vi "Posterior_LDA_maker.vi"(2 "Target_LDA_Parameter":dbl[][](array[numeric]), 3 "Nontarget_LDA_Parameter":dbl[][](array[numeric])) -> (0 "A * B 2":T1 caption="A * B(Point)", 1 "A * B":T1 caption="A * B(Matrix)")   [LabVIEW 2013]
uses:
  <vilib>/Analysis/Matrix/Datatypes/RealMatrix.ctl
  <vilib>/Analysis/baseanly.llb/Mean (DBL).vi
  <vilib>/Analysis/baseanly.llb/Real A x B.vi
  <vilib>/Analysis/7linalg.llb/Real Transpose Matrix.vi
  <vilib>/Analysis/Matrix/Numeric/Conversions/Array To Matrix - RA2.vi
  <vilib>/Analysis/Matrix/Numeric/Multiply/Multiply - RM,R.vi
  <vilib>/Analysis/Matrix/Numeric/Add/Add - RM,RM.vi
  <vilib>/Analysis/baseanly.llb/Real Inverse Matrix.vi
  <vilib>/Analysis/Matrix/Numeric/Conversions/Array To Matrix - RA.vi
  <vilib>/Analysis/Matrix/Numeric/Subtract/Subtract - RM,RM.vi
  <vilib>/Analysis/Matrix/Numeric/Multiply/Multiply - R,RM.vi
  <vilib>/Analysis/Matrix/Numeric/Multiply/Multiply - RM,RM.vi
  <vilib>/Analysis/NI_AALBase.lvlib
  <vilib>/Analysis/Matrix/NI_Matrix.lvlib
  <vilib>/Analysis/NI_AALPro.lvlib
panel:
  out "Array":dbl[](array[numeric])
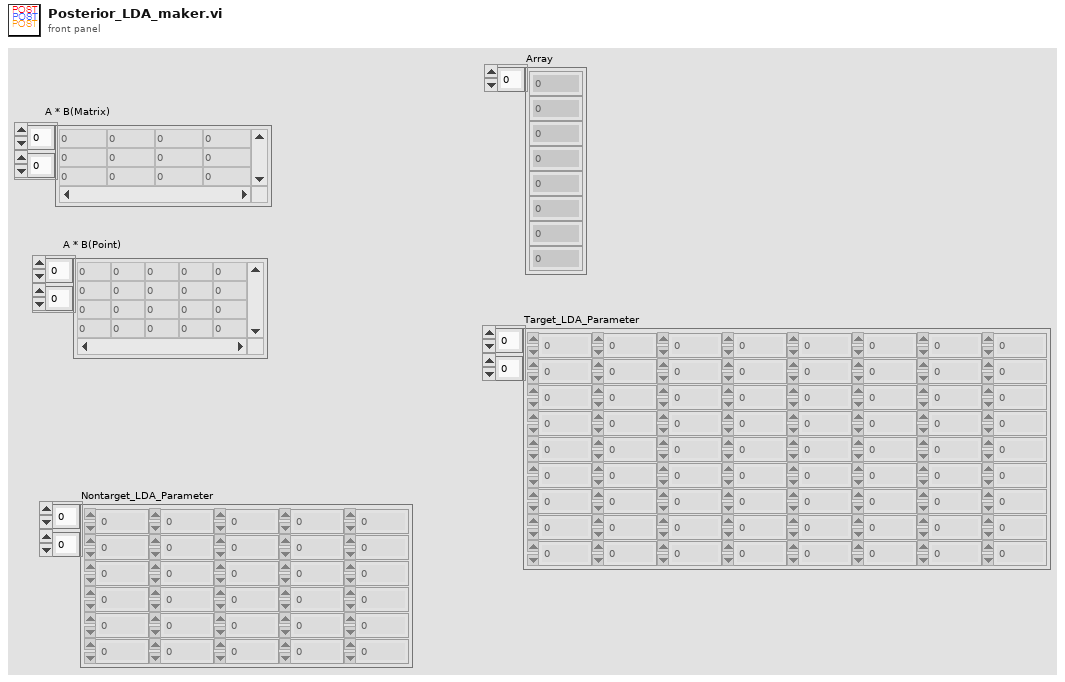
[diagram p1: front panel]
types:
  T1 = typedef "NI_Matrix.lvlib/RealMatrix.ctl" = dbl[][]
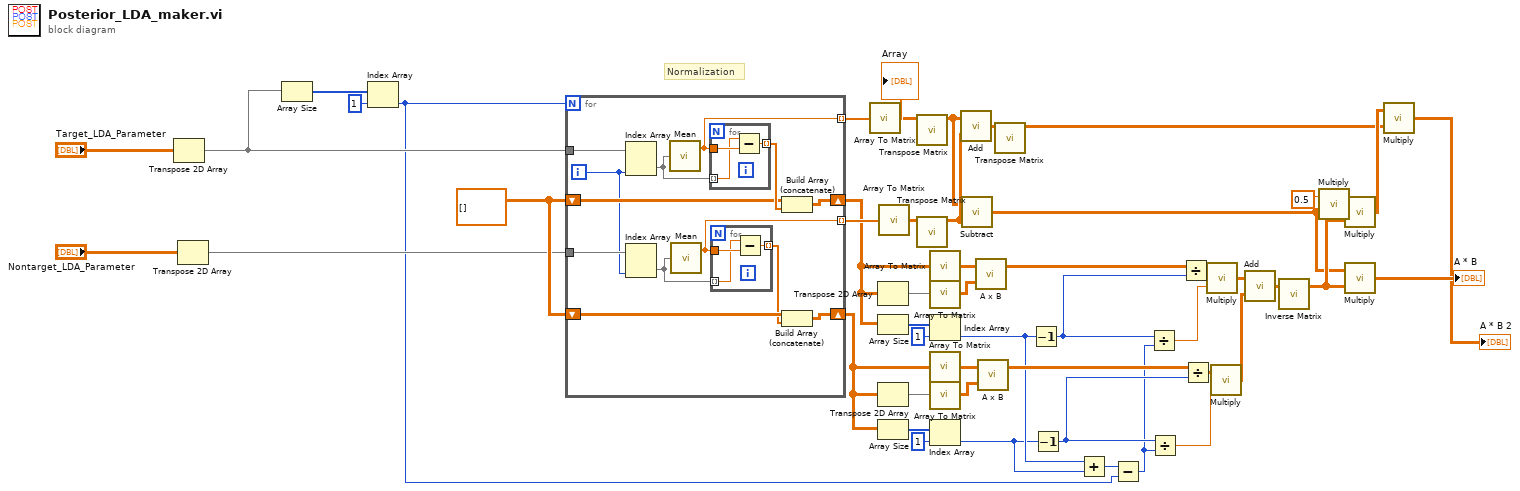
[diagram p0: block diagram]
diagram:
  w49 = dbl[][] []
  # "Normalization"
  n1 = Transpose 2D Array(2D array="Target_LDA_Parameter") -> (transposed array=w3:dbl[][])
  n2 = Transpose 2D Array(2D array="Nontarget_LDA_Parameter") -> (transposed array=w2:dbl[][])
  n3 = Array Size(array=w3) -> (size(s)=w5:i32[])
  n4 = Index Array(array=w5, index=1) -> (element=w1:i32)
  n5 = for {
    N: w1 -> [_]
    shift-right: [w62] -> w36
    shift-left: w49 -> [w61]
    shift-right: [w59] -> w34
    shift-left: w49 -> [w60]
    tunnel: [w57] -> w48 mode=indexing
    tunnel: [w56] -> w47 mode=indexing
    tunnel: w3 -> [w55]
    tunnel: w2 -> [w54]
    i -> [w51]
    n6 = Index Array(array=w55, index (col)=w51) -> (element=w53:dbl[])  [unwired: 1 in]
    n7 = Index Array(array=w54, index (col)=w51) -> (element=w52:dbl[])  [unwired: 1 in]
    n8 = call-poly <vilib>:"Mean.vi"("X"=w53) -> ("mean"=w57:dbl)  [unwired: 1 out]
    n9 = call-poly <vilib>:"Mean.vi"("X"=w52) -> ("mean"=w56:dbl)  [unwired: 1 out]
    n10 = for {
      tunnel: w57 -> [w69]
      tunnel: [w68] -> w63 mode=indexing
      tunnel: w53 -> [w67] mode=indexing
      n11 = Subtract(x=w67, y=w69) -> (x-y=w68:dbl)
    }
    n12 = for {
      tunnel: w56 -> [w66]
      tunnel: [w65] -> w58 mode=indexing
      tunnel: w52 -> [w64] mode=indexing
      n13 = Subtract(x=w64, y=w66) -> (x-y=w65:dbl)
    }
    n14 = Build Array (concatenate)(w61, w63) -> (w62:dbl[][])
    n15 = Build Array (concatenate)(w60, w58) -> (w59:dbl[][])
  }
  "Array" <- w48
  n16 = call-poly <vilib>:"Array To Matrix.vi"("Real 1D Array"=w48) -> ("Real Matrix (Column Vector)"=w46:T1)
  n17 = Transpose 2D Array(2D array=w36) -> (transposed array=w37:dbl[][])
  n18 = Array Size(array=w36) -> (size(s)=w38:i32[])
  n19 = Transpose 2D Array(2D array=w34) -> (transposed array=w35:dbl[][])
  n20 = Array Size(array=w34) -> (size(s)=w41:i32[])
  n21 = call-poly <vilib>:"Array To Matrix.vi"("Real 1D Array"=w47) -> ("Real Matrix (Column Vector)"=w45:T1)
  n22 = call-poly <vilib>:"Transpose Matrix.vi"("Input Matrix"=w46) -> ("Matrix Transpose"=w43:T1)  [unwired: 9 in, 1 out]
  n23 = call-poly <vilib>:"Transpose Matrix.vi"("Input Matrix"=w45) -> ("Matrix Transpose"=w44:T1)  [unwired: 9 in, 1 out]
  n24 = call-poly <vilib>:"Array To Matrix.vi"("Real 2D Array"=w36) -> ("Real Matrix"=w33:T1)
  n25 = call-poly <vilib>:"Array To Matrix.vi"("Real 2D Array"=w37) -> ("Real Matrix"=w32:T1)
  n26 = Index Array(array=w38, index=1) -> (element=w27:i32)
  n27 = call-poly <vilib>:"Array To Matrix.vi"("Real 2D Array"=w34) -> ("Real Matrix"=w31:T1)
  n28 = call-poly <vilib>:"Array To Matrix.vi"("Real 2D Array"=w35) -> ("Real Matrix"=w30:T1)
  n29 = Index Array(array=w41, index=1) -> (element=w26:i32)
  n30 = call-poly <vilib>:"Add.vi"("Real Matrix B"=w44, "Real Matrix A"=w43) -> ("A + B"=w42:T1)
  n31 = call-poly <vilib>:"Subtract.vi"("Real Matrix B"=w44, "Real Matrix A"=w43) -> ("A - B"=w7:T1)
  n32 = call-poly <vilib>:"A x B.vi"("B"=w32, "A"=w33) -> ("A x B"=w29:T1)  [unwired: 1 out]
  n33 = call-poly <vilib>:"A x B.vi"("B"=w30, "A"=w31) -> ("A x B"=w28:T1)  [unwired: 1 out]
  n34 = call-poly <vilib>:"Transpose Matrix.vi"("Input Matrix"=w42) -> ("Matrix Transpose"=w8:T1)  [unwired: 9 in, 1 out]
  n35 = Decrement(x=w27) -> (x-1=w24:i32)
  n36 = Decrement(x=w26) -> (x-1=w23:i32)
  n37 = Add(x=w27, y=w26) -> (x+y=w25:i32)
  n38 = Subtract(x=w25, y=w1) -> (x-y=w22:i32)
  n39 = Divide(x=w24, y=w22) -> (x/y=w20:dbl)
  n40 = Divide(x=w23, y=w22) -> (x/y=w18:dbl)
  n41 = Divide(x=w29, y=w24) -> (x/y=w21:T1)
  n42 = Divide(x=w28, y=w23) -> (x/y=w19:T1)
  n43 = call-poly <vilib>:"Multiply.vi"("Real Scalar c"=w20, "Real Matrix A"=w21) -> ("A * c"=w17:T1)
  n44 = call-poly <vilib>:"Multiply.vi"("Real Scalar c"=w18, "Real Matrix A"=w19) -> ("A * c"=w16:T1)
  n45 = call-poly <vilib>:"Add.vi"("Real Matrix B"=w16, "Real Matrix A"=w17) -> ("A + B"=w15:T1)
  n46 = call-poly <vilib>:"Inverse Matrix.vi"("Input Matrix"=w15) -> ("Inverse Matrix"=w12:T1)  [unwired: 1 in, 1 out]
  n47 = call-poly <vilib>:"Multiply.vi"("Real Matrix A"=w7, "Real Scalar c"=0.5) -> ("c * A"=w13:T1)
  n48 = call-poly <vilib>:"Multiply.vi"("Real Matrix B"=w12, "Real Matrix A"=w13) -> ("A * B"=w11:T1)
  n49 = call-poly <vilib>:"Multiply.vi"("Real Matrix B"=w12, "Real Matrix A"=w7) -> ("A * B"=→"A * B":T1)
  n50 = call-poly <vilib>:"Multiply.vi"("Real Matrix B"=w8, "Real Matrix A"=w11) -> ("A * B"=→"A * B 2":T1)
